vi "1_While_loop.vi"() -> ()   [LabVIEW 2019]
panel:
  out "Wartość\ndekrementowana":dbl
  in  "Wartość\npoczątkowa":dbl=20.0 min=0.0 step=1.0
  in  "Opóźnienie pętli [s]":dbl=0.1 caption="Delay Time (s)" min=0.0 step=0.1 format="%#.2g"
  out "Liczba \nwykonanych iteracji":dbl
  in  "?":bool
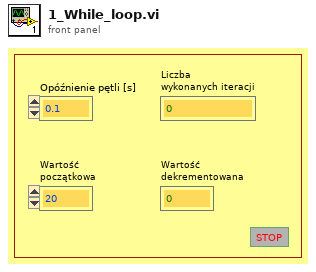
[diagram p1: front panel]
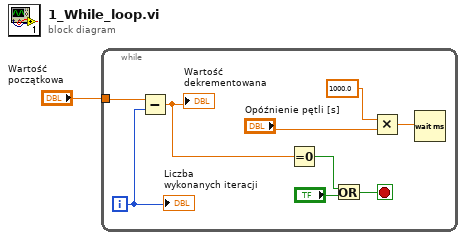
[diagram p0: block diagram]
diagram:
  n1 = while {
    tunnel: "Wartość\npoczątkowa" -> [w6]
    i -> [w5]
    stop <- w9 stop-if-true
    n2 = Subtract(x=w6, y=w5) -> (x-y=w7:dbl)
    "Wartość\ndekrementowana" <- w7
    n3 = Equal To 0?(x=w7) -> (x = 0?=w8:bool)
    n4 = Or(x=w8, y="?") -> (x .or. y?=w9:bool)
    n5 = Multiply(x=1000.0, y="Opóźnienie pętli [s]") -> (x*y=w4:dbl)
    n6 = Wait (ms)(milliseconds to wait=w4) -> ()  [unwired: 1 out]
    "Liczba \nwykonanych iteracji" <- w5
  }
